vi "TranslateGrpcError.vi"(8 "error in":errorcluster, 10 "Error Message":string, 11 "Error Code":i32) -> (0 "error out":errorcluster)   [LabVIEW 2019, in "grpc-lvsupport.lvlib"]
uses:
  grpc-lvsupport.lvlib
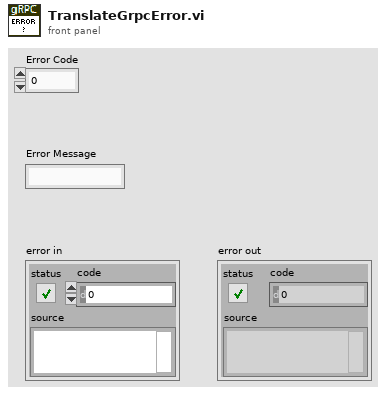
[diagram p1: front panel]
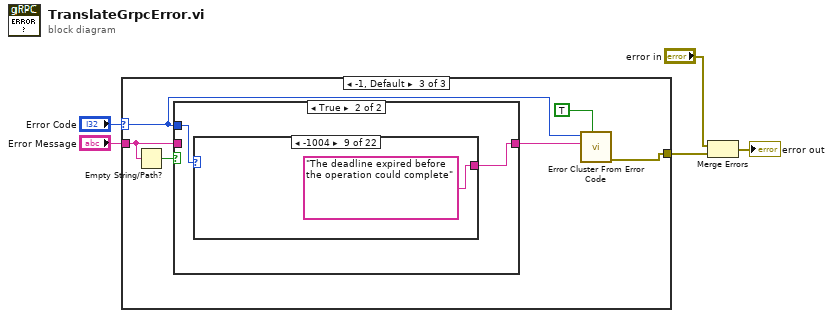
[diagram p0: block diagram]
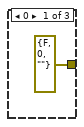
[diagram p2: hidden frame]
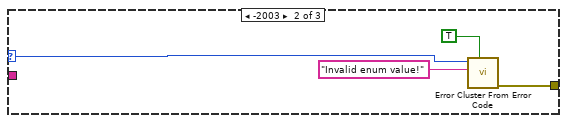
[diagram p3: hidden frame]
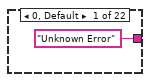
[diagram p5: hidden frame]
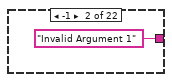
[diagram p6: hidden frame]
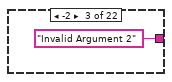
[diagram p7: hidden frame]
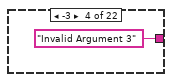
[diagram p8: hidden frame]
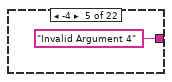
[diagram p9: hidden frame]
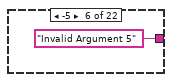
[diagram p10: hidden frame]
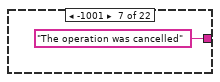
[diagram p11: hidden frame]
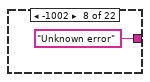
[diagram p12: hidden frame]
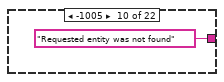
[diagram p13: hidden frame]
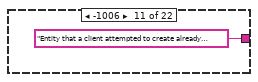
[diagram p14: hidden frame]
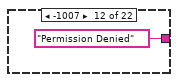
[diagram p15: hidden frame]
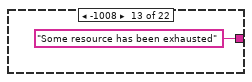
[diagram p16: hidden frame]
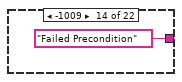
[diagram p17: hidden frame]
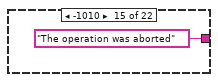
[diagram p18: hidden frame]
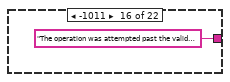
[diagram p19: hidden frame]
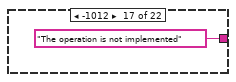
[diagram p20: hidden frame]
diagram:
  n1 = case shown="-1, Default" "Error Code" {
    selector: "Error Code" -> [_ w8 w13]
    tunnel: [errorcluster {"status"=FALSE, "code"=0, "source"=""} ("error out") w7 w11] -> w4
    tunnel: "Error Message" -> [_ _ w15]
    frame 0 {
    }
    frame -2003 {
      n2 = call <vilib>:"Error Cluster From Error Code.vi"("show call chain? (False)"=TRUE, "error message (\"\")"="Invalid enum value!" ("error source (\" \")"), "error code (0)"=w8) -> ("error out"=w7:errorcluster)  [unwired: 6 in]
    }
    frame -1, Default {
      n3 = Empty String/Path?(string/path=w15) -> (empty?=w16:bool)
      n4 = case shown="True" w16 {
        tunnel: w13 -> [_ w19]
        tunnel: [w17 w18] -> w14
        tunnel: w15 -> [w17 _]
        frame False {
        }
        frame True {
          n5 = case shown="-1004" w19 {
            tunnel: ["Unknown Error" "Invalid Argument 1" "Invalid Argument 2" "Invalid Argument 3" "Invalid Argument 4" "Invalid Argument 5" "The operation was cancelled" "Unknown error" "The deadline expired before the operation could complete" "Requested entity was not found" "Entity that a client attempted to create already exists" "Permission Denied" "Some resource has been exhausted" "Failed Precondition" "The operation was aborted" "The operation was attempted past the valid range" "The operation is not implemented" "\tInternal error" "The service is currently unavailable" "Unrecoverable data loss or corruption" "The request does not have valid authentication credentials" "The client specified an invalid argument"] -> w18
            frame 0, Default {
            }
            frame -1 {
            }
            frame -2 {
            }
            frame -3 {
            }
            frame -4 {
            }
            frame -5 {
            }
            frame -1001 {
            }
            frame -1002 {
            }
            frame -1004 {
            }
            frame -1005 {
            }
            frame -1006 {
            }
            frame -1007 {
            }
            frame -1008 {
            }
            frame -1009 {
            }
            frame -1010 {
            }
            frame -1011 {
            }
            frame -1012 {
            }
            frame -1013 {
            }
            frame -1014 {
            }
            frame -1015 {
            }
            frame -1016 {
            }
            frame -1003 {
            }
          }
        }
      }
      n6 = call <vilib>:"Error Cluster From Error Code.vi"("show call chain? (False)"=TRUE, "error message (\"\")"=w14, "error code (0)"=w13) -> ("error out"=w11:errorcluster)  [unwired: 6 in]
    }
  }
  n7 = Merge Errors("error in", w4) -> (→"error out":errorcluster)
